vi "GatedTrig.vi"(0 "reference":refnum<k24>, 11 "error in (no error)":errorcluster) -> (1 "HighThreshold":dbl, 2 "WindowTop":dbl, 3 "Hysteresis":i32(ring) items=["Negative", "Positive"], 4 "reference out":refnum<k24>, 6 "AnalogLevel":dbl, 7 "When":i32(ring) items=["InsideWindow", "OutsideWindow"], 8 "DigitalLevel":i32(ring) items=["GateHigh", "GateLow"], 10 "Type":i32(ring) items=["None", "AnalogLevel", "DigitalLevel", "AnalogHysteresis", "AnalogWindow"], 12 "LowThreshold":dbl, 13 "WindowBottom":dbl, 14 "Position":i32(ring) items=["GateAbove", "GateBelow"], 15 "error out":errorcluster)   [LabVIEW 2009]
uses:
  C:/Program Files/National Instruments/LabVIEW 2009/vi.lib/ULx/ULx_LV.dll
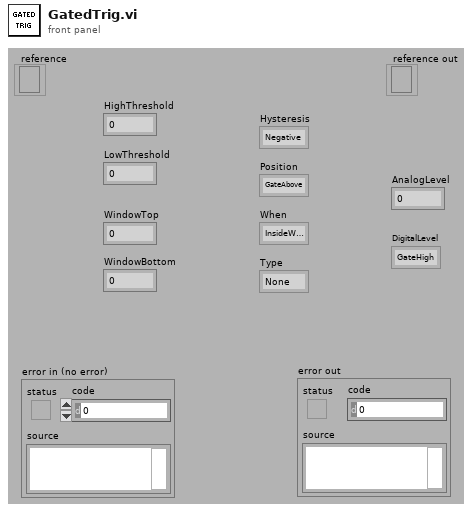
[diagram p1: front panel]
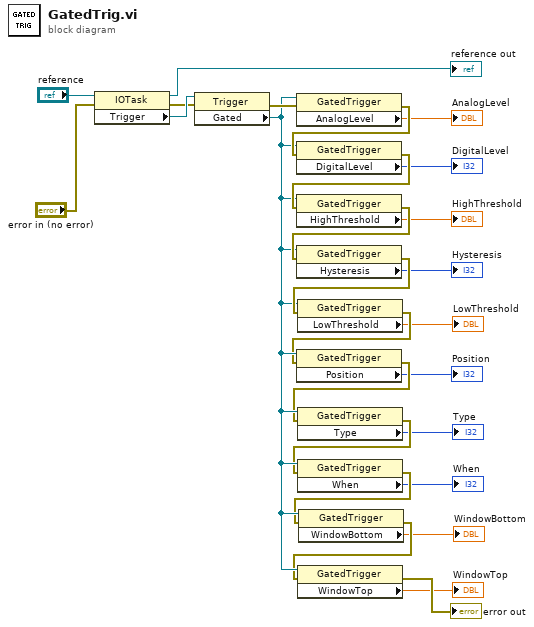
[diagram p0: block diagram]
diagram:
  n1 = property class="IOTask"(reference="reference", error in="error in (no error)") -> (reference out=→"reference out":refnum<k24>, error out=w26:errorcluster, "Trigger"=w27:refnum<k24>)
  n2 = property class="Trigger"(reference=w27, error in=w26) -> (error out=w25:errorcluster, "Gated"=w20:refnum<k24>)  [unwired: 1 out]
  n3 = property class="GatedTrigger"(reference=w20, error in=w25) -> (error out=w24:errorcluster, "AnalogLevel"=→"AnalogLevel":dbl)  [unwired: 1 out]
  n4 = property class="GatedTrigger"(reference=w20, error in=w24) -> (error out=w23:errorcluster, "DigitalLevel"=→"DigitalLevel":i32)  [unwired: 1 out]
  n5 = property class="GatedTrigger"(reference=w20, error in=w23) -> (error out=w22:errorcluster, "HighThreshold"=→"HighThreshold":dbl)  [unwired: 1 out]
  n6 = property class="GatedTrigger"(reference=w20, error in=w22) -> (error out=w21:errorcluster, "Hysteresis"=→"Hysteresis":i32)  [unwired: 1 out]
  n7 = property class="GatedTrigger"(reference=w20, error in=w21) -> (error out=w19:errorcluster, "LowThreshold"=→"LowThreshold":dbl)  [unwired: 1 out]
  n8 = property class="GatedTrigger"(reference=w20, error in=w19) -> (error out=w18:errorcluster, "Position"=→"Position":i32)  [unwired: 1 out]
  n9 = property class="GatedTrigger"(reference=w20, error in=w18) -> (error out=w17:errorcluster, "Type"=→"Type":i32)  [unwired: 1 out]
  n10 = property class="GatedTrigger"(reference=w20, error in=w17) -> (error out=w16:errorcluster, "When"=→"When":i32)  [unwired: 1 out]
  n11 = property class="GatedTrigger"(reference=w20, error in=w16) -> (error out=w15:errorcluster, "WindowBottom"=→"WindowBottom":dbl)  [unwired: 1 out]
  n12 = property class="GatedTrigger"(reference=w20, error in=w15) -> (error out=→"error out":errorcluster, "WindowTop"=→"WindowTop":dbl)  [unwired: 1 out]
